vi "LDT Parse XML Locutus Obs Status.vi"(11 "XML String":string) -> (3 "FITS Keyword":T1)   [LabVIEW 2022 SP3, in "LDT Telescope.lvclass"]
uses:
  LDT Telescope.lvclass
  LDT FITS Keyword cluster.ctl
  LDT Telescope.lvclass/LDT Telescope.ctl
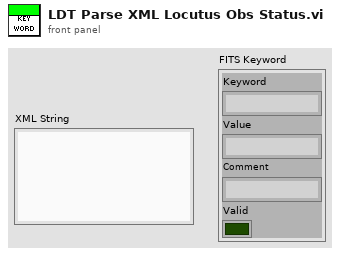
[diagram p1: front panel]
types:
  T1 = typedef "LDT Telescope.lvclass/LDT FITS Keyword cluster.ctl" = cluster{"Keyword":string, "Value":string, "Comment":string, "Valid":bool}
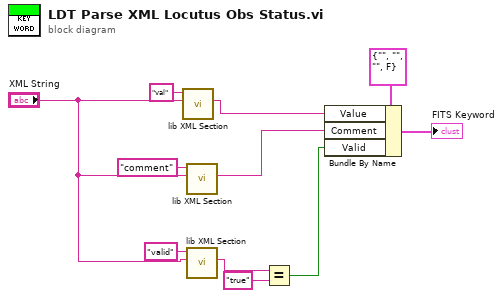
[diagram p0: block diagram]
diagram:
  n1 = call "lib XML Section.vi"("XML String"="XML String", "XML Topic"="val") -> ("XML Topic Body"=w4:string)  [unwired: 6 in, 3 out]
  n2 = call "lib XML Section.vi"("XML String"="XML String", "XML Topic"="comment") -> ("XML Topic Body"=w3:string)  [unwired: 6 in, 3 out]
  n3 = call "lib XML Section.vi"("XML String"="XML String", "XML Topic"="valid") -> ("XML Topic Body"=w7:string)  [unwired: 6 in, 3 out]
  n4 = Equal?(x=w7, y="true") -> (x = y?=w2:bool)
  n5 = Bundle By Name(cluster=T1 {"Keyword"="", "Value"="", "Comment"="", "Valid"=FALSE} ("FITS Keyword"), "Value"=w4, "Comment"=w3, "Valid"=w2) -> (→"FITS Keyword":T1)
